vi "Configure Modulation (ASK).vi"(5 "Channel (1:Channel 1)":i32(ring)=1 items=["Channel 1"=1, "Channel 2"=2], 7 "Enable ASK Modulation (T:Enable)":bool=TRUE, 8 "error in (no error)":errorcluster, 9 "Key Frequency (100.000 Hz)":dbl=100.0 format="%.3f", 10 "ASK Source (0: Internal)":u16(ring) items=["Internal", "External"], 11 "VISA resource name":refnum<visa-resource-name>) -> (0 "error out":errorcluster, 3 "VISA resource name out":refnum<visa-resource-name>)   [LabVIEW 2015, in "SDG X Series.lvlib"]
doc: "Configures and enables ASK modulation.\n\n<B>Note:</B> The carrier waveform shape and parameters are set by the Configure Standard Waveform VI."
uses:
  <instrlib>/SDG X Series/SDG X Series.lvlib
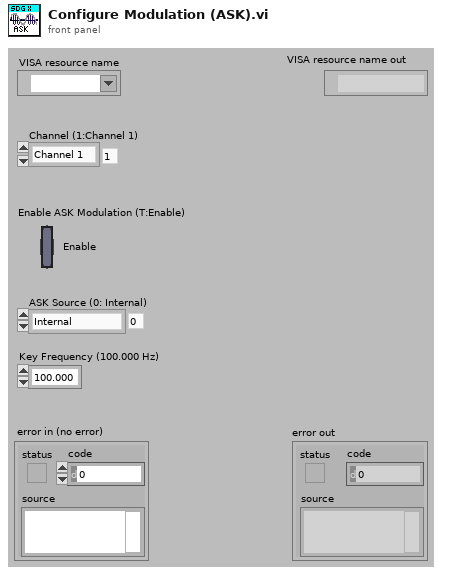
[diagram p1: front panel]
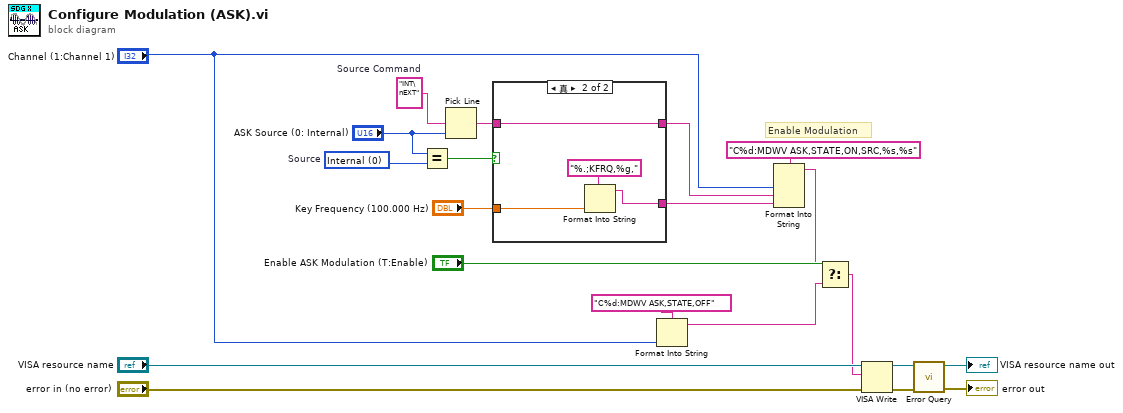
[diagram p0: block diagram]
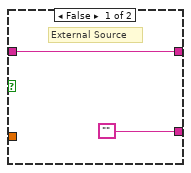
[diagram p2: hidden frame]
diagram:
  w14 = "INT\nEXT"  # Source Command
  w10 = u16 0 items=["Internal", "External"]  # Source
  # "Enable Modulation"
  n1 = Equal?(x="ASK Source (0: Internal)", y=w10) -> (x = y?=w13:bool)
  n2 = Pick Line(multi-line string=w14, line index="ASK Source (0: Internal)") -> (output string=w12:string)  [unwired: 1 in]
  n3 = case shown="真" w13 {
    tunnel: w12 -> [w23 w27]
    tunnel: [w23 w27] -> w8
    tunnel: ["" w24] -> w7
    tunnel: "Key Frequency (100.000 Hz)" -> [_ w25]
    frame False {
      # "External Source"
    }
    frame True {
      n4 = Format Into String(format string="%.;KFRQ,%g,", w25) -> (resulting string=w24:string)  [unwired: 2 in, 1 out]
    }
  }
  n5 = Format Into String(format string="C%d:MDWV ASK,STATE,OFF", "Channel (1:Channel 1)") -> (resulting string=w3:string)  [unwired: 2 in, 1 out]
  n6 = Format Into String(format string="C%d:MDWV ASK,STATE,ON,SRC,%s,%s", "Channel (1:Channel 1)", w8, w7) -> (resulting string=w4:string)  [unwired: 2 in, 1 out]
  n7 = Select(t=w4, s="Enable ASK Modulation (T:Enable)", f=w3) -> (s? t:f=w2:string)
  n8 = VISA Write(VISA resource name="VISA resource name", write buffer=w2, error in (no error)="error in (no error)") -> (VISA resource name out=w19:refnum<visa-resource-name>, error out=w18:errorcluster)  [unwired: 1 out]
  n9 = call <instrlib>:"Error Query.vi"("error in (no error)"=w18, "VISA resource name"=w19) -> ("error out"=→"error out":errorcluster, "VISA resource name out"=→"VISA resource name out":refnum<visa-resource-name>)  [unwired: 6 in, 2 out]
